vi "Configure Resolution and Video Bandwidth.vi"(8 "error in (no error)":errorcluster, 9 "VBW [Hz]":dbl, 10 "RBW [Hz]":dbl, 11 "MXA in":refnum<class "MXA.lvclass">) -> (0 "error out":errorcluster, 3 "MXA out":refnum<class "MXA.lvclass">)   [LabVIEW 2020, in "MXA.lvclass"]
uses:
  MXA.lvclass
  C:/Sandbox/Git_Sandbox/WiSpry Test Framework source code (LV20)/WiSpry Test Framework/Instruments/Instrument.lvclass
  C:/Sandbox/Git_Sandbox/WiSpry Test Framework source code (LV20)/WiSpry Test Framework/Instruments/Spectrum Analyzer/Spectrum Analyzer.lvclass
  Instrument.lvclass/Instrument.ctl
  Spectrum Analyzer.lvclass/Spectrum Analyzer.ctl
  Instrument.lvclass
  Spectrum Analyzer.lvclass
  <instrlib>/Agilent MXA Series/Agilent MXA Series.lvlib
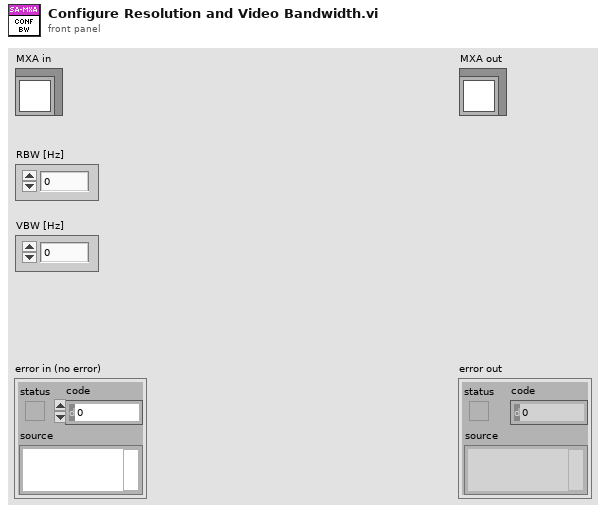
[diagram p1: front panel]
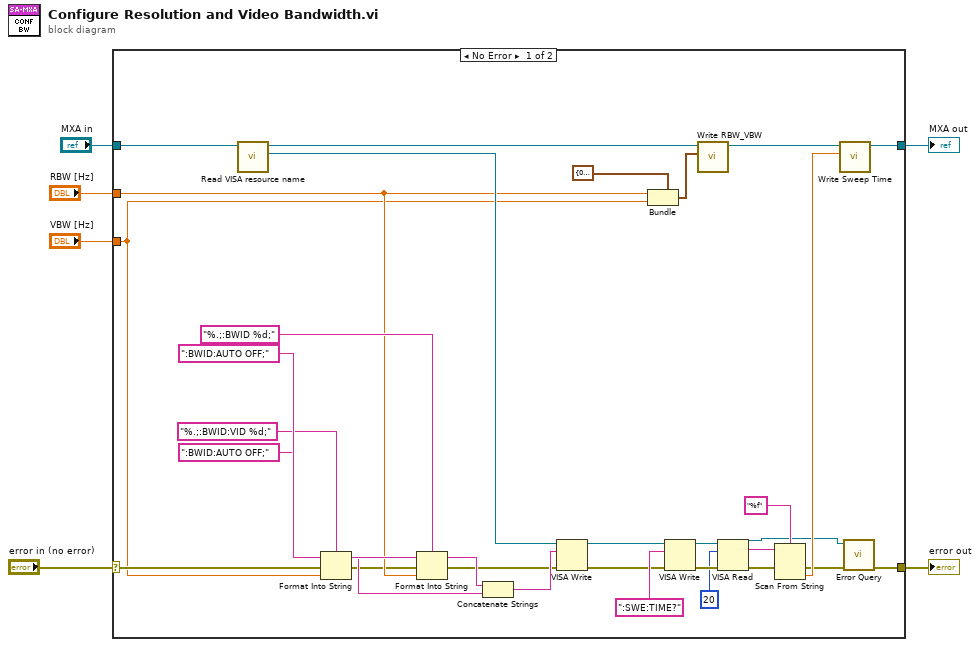
[diagram p0: block diagram]
diagram:
  n1 = case shown="No Error" "error in (no error)" {
    selector: "error in (no error)" -> [w38 w40]
    tunnel: "MXA in" -> [w36 w39]
    tunnel: [w7 w40] -> w4
    tunnel: [w31 w39] -> w3
    tunnel: "VBW [Hz]" -> [w17 _]
    tunnel: "RBW [Hz]" -> [w18 _]
    frame No Error {
      n2 = call "Read VISA resource name.vi"("Instrument in"=w36) -> ("VISA resource name"=w37:refnum<visa-resource-name>, "Instrument out"=w35:refnum<class "MXA.lvclass">)  [unwired: 9 in]
      n3 = Format Into String(format string="%.;:BWID:VID %d;", initial string=":BWID:AUTO OFF;" ("format string"), error in=w38, w17) -> (resulting string=w15:string, error out=w11:errorcluster)
      n4 = Format Into String(format string="%.;:BWID %d;", initial string=":BWID:AUTO OFF;" ("format string"), error in=w11, w18) -> (resulting string=w16:string, error out=w10:errorcluster)
      n5 = Concatenate Strings(w16, w15) -> (w12:string)
      n6 = VISA Write(VISA resource name=w37, write buffer=w12, error in (no error)=w10) -> (VISA resource name out=w13:refnum<visa-resource-name>, error out=w14:errorcluster)  [unwired: 1 out]
      n7 = Bundle(cluster=cluster{"RBW":dbl, "VBW":dbl} {"RBW"=0.0, "VBW"=0.0} ("RBW/VBW"), "RBW"=w18, "VBW"=w17) -> (w33:cluster{"RBW":dbl, "VBW":dbl})
      n8 = VISA Write(VISA resource name=w13, write buffer=":SWE:TIME?", error in (no error)=w14) -> (VISA resource name out=w30:refnum<visa-resource-name>, error out=w29:errorcluster)  [unwired: 1 out]
      n9 = call "Write RBW_VBW.vi"("RBW/VBW"=w33, "Spectrum Analyzer in"=w35) -> ("Spectrum Analyzer out"=w32:refnum<class "MXA.lvclass">)  [unwired: 9 in]
      n10 = VISA Read(VISA resource name=w30, byte count=u32 20, error in (no error)=w29) -> (VISA resource name out=w8:refnum<visa-resource-name>, read buffer=w25:string, error out=w26:errorcluster)  [unwired: 1 out]
      n11 = Scan From String(format string="%f", input string=w25, error in=w26) -> (error out=w9:errorcluster, output 1=w23:dbl)  [unwired: 2 in, 2 out]
      n12 = call "Write Sweep Time.vi"("Sweep Time"=w23, "Spectrum Analyzer in"=w32) -> ("Spectrum Analyzer out"=w31:refnum<class "MXA.lvclass">)  [unwired: 9 in]
      n13 = call <instrlib>:"Error Query.vi"("error in (no error)"=w9, "VISA resource name"=w8) -> ("error out"=w7:errorcluster)  [unwired: 6 in, 3 out]
    }
    frame Error {
    }
  }
  "error out" <- w4
  "MXA out" <- w3
